vi "Alphabetize Cluster Control.vi"(8 "Error In":errorcluster) -> (0 "Error Out":errorcluster)   [LabVIEW 2017, in "Tests.lvlib" / "Toolkit.lvlib"]
uses:
  Toolkit.lvlib
  <vilib>/Utility/traverseref.llb/TRef TravTarget.ctl
  <vilib>/addons/_JKI Toolkits/Caraya/classes/Test/Test.lvclass
  src/Toolkit/Toolkit.lvlib
  <vilib>/Utility/traverseref.llb/VI Scripting - Traverse.lvlib
  <vilib>/addons/_JKI Toolkits/Caraya/classes/Assert/Assert.lvclass
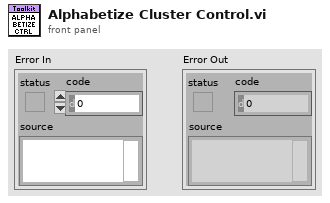
[diagram p1: front panel]
types:
  T1 = typedef "TRef TravTarget.ctl" = enum16{"FP", "BD", "Other"}
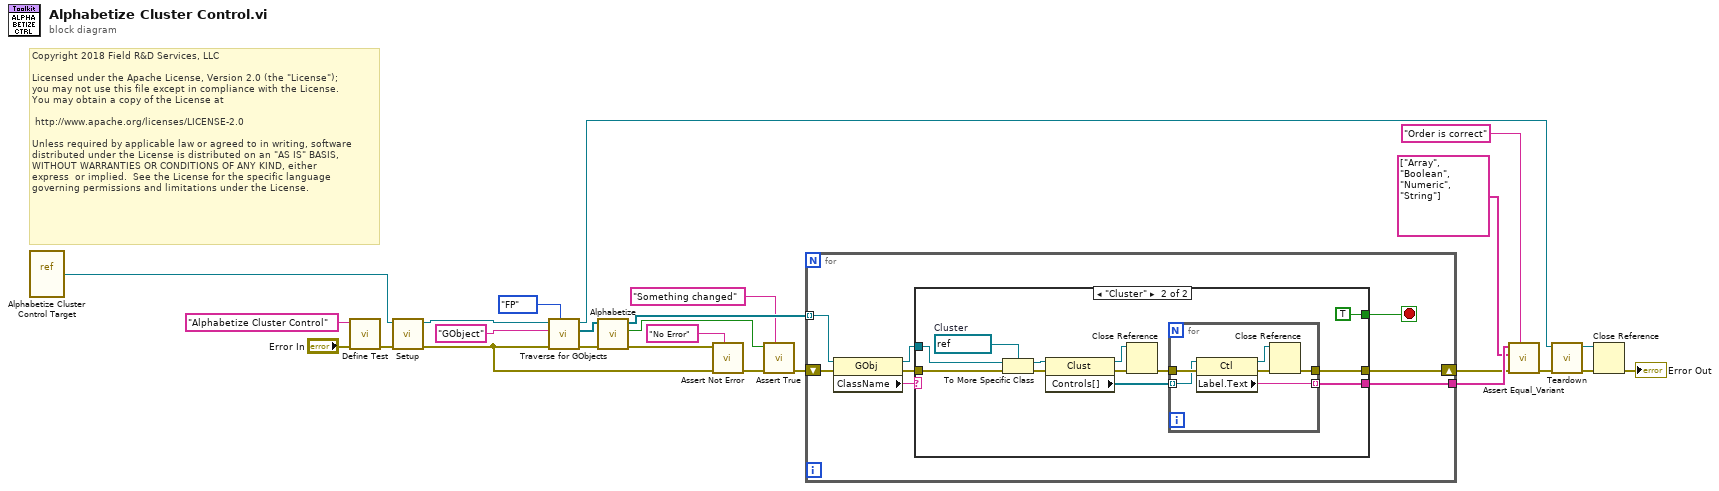
[diagram p0: block diagram]
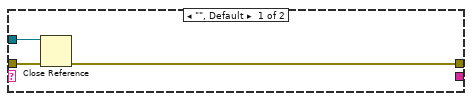
[diagram p2: hidden frame]
diagram:
  # "Copyright 2018 Field R&D Services, LLC\n\nLicensed under the Apache License, Version 2.0 (the \"License\");\nyou may not use this file except in compliance with the License.\nYou may obtain a copy of the License at\n\n\thttp://www.apache.org/licenses/LICENSE-2.0\n\nUnless required by applicable law or agreed to in writing, software\ndistributed under the License is distributed on an \"AS IS\" BASIS,\nWITHOUT WARRANTIES OR CONDITIONS OF ANY KIND, either \nexpress  or implied.  See the License for the specific language \ngoverning permissions and limitations under the License."
  n1 = vi-ref "Alphabetize Cluster Control Target.vi"() -> (w23:refnum<vi>)
  n2 = call <vilib>:"Define Test.vi"("error in (no error)"="Error In", "Label (VI Title)"="Alphabetize Cluster Control") -> ("error out"=w24:errorcluster)  [unwired: 9 in]
  n3 = call "Setup.vi"("Error In"=w24, "VI In"=w23) -> ("Error Out"=w12:errorcluster, "VI Out"=w21:refnum<vi>)  [unwired: 8 in]
  n4 = call <vilib>:"Traverse for GObjects.vi"("Traverse Target"=TRef_TravTarget."FP", "error in (no error)"=w12, "Class Name"="GObject", "VI Refnum"=w21) -> ("error out"=w5:errorcluster, "References"=w6:refnum<vi>[], "dup VI Refnum"=w10:refnum<vi>)  [unwired: 4 in, 1 out]
  n5 = call "Alphabetize.vi"("Error In"=w5, "Clusters In"=w6) -> ("Error Out"=w15:errorcluster, "Change?"=w2:bool, "Clusters Out"=w4:refnum<vi>[])  [unwired: 7 in]
  n6 = call <vilib>:"Assert Not Error.vi"("Label"="No Error", "error in (no error)"=w12, "Not Error?"=w15) -> ("error out"=w14:errorcluster)  [unwired: 8 in]
  n7 = call <vilib>:"Assert True.vi"("Label"="Something changed", "error in (no error)"=w14, "True?"=w2) -> ("error out"=w3:errorcluster)  [unwired: 8 in]
  n8 = for {
    tunnel: [w34] -> w19
    shift-right: [w32] -> w13
    shift-left: w3 -> [w33]
    tunnel: w4 -> [w30] mode=indexing
    stop <- w28 stop-if-true
    n9 = property class="GObj"(reference=w30, error in=w33) -> (reference out=w27:refnum<vi>, error out=w31:errorcluster, "ClassName"=w29:string)
    n10 = case shown="\"Cluster\"" w29 {
      tunnel: [_ w45] -> w34
      tunnel: [w35 w44] -> w32
      tunnel: w31 -> [w36 w43]
      tunnel: [_ TRUE] -> w28
      tunnel: w27 -> [w37 w40]
      frame "", Default {
        n11 = Close Reference(reference=w37, error in (no error)=w36) -> (error out=w35:errorcluster)
      }
      frame "Cluster" {
        w39 = refnum<vi> refnum  # Cluster
        n12 = To More Specific Class(target class=w39, reference=w40, error in=w43) -> (specific class reference=w38:refnum<vi>, error out=w41:errorcluster)
        n13 = property class="Clust"(reference=w38, error in=w41) -> (reference out=w46:refnum<vi>, error out=w48:errorcluster, "Controls[]"=w49:refnum<vi>[])
        n14 = Close Reference(reference=w46, error in (no error)=w48) -> (error out=w47:errorcluster)
        n15 = for {
          tunnel: w49 -> [w50] mode=indexing
          tunnel: w47 -> [w55]
          tunnel: [w54] -> w45 mode=indexing
          tunnel: [w51] -> w44
          n16 = property class="Ctl"(reference=w50, error in=w55) -> (reference out=w52:refnum<vi>, error out=w53:errorcluster, "Label.Text"=w54:string)
          n17 = Close Reference(reference=w52, error in (no error)=w53) -> (error out=w51:errorcluster)
        }
      }
    }
  }
  n18 = call <vilib>:"Assert Equal_Variant.vi"("Label"="Order is correct", "error in (no error)"=w13, "Y"=string[] ["Array", "Boolean", "Numeric", "String"], "X"=w19) -> ("error out"=w11:errorcluster)  [unwired: 7 in]
  n19 = call "Teardown.vi"("Error In"=w11, "VI In"=w10) -> ("Error Out"=w8:errorcluster, "VI Out"=w9:refnum<vi>)  [unwired: 8 in]
  n20 = Close Reference(reference=w9, error in (no error)=w8) -> (error out=→"Error Out":errorcluster)
